vi "x_axisPID_ALB.vi"(6 "First Call?: T/F":bool, 10 "x axis":dbl) -> (2 "x axis out":dbl)   [LabVIEW 2017]
uses:
  <vilib>/addons/control/pid/NI_PID_pid.lvlib
  <vilib>/addons/control/pid/pid.llb/PID (DBL).vi
  <vilib>/addons/control/pid/pid.llb/PID Output Rate Limiter (DBL).vi
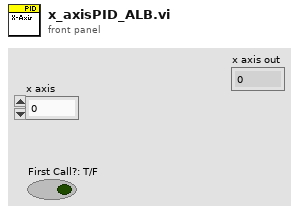
[diagram p1: front panel]
types:
  T1 = cluster{"P":dbl, "I":dbl, "derivative time (Td, min)":dbl}
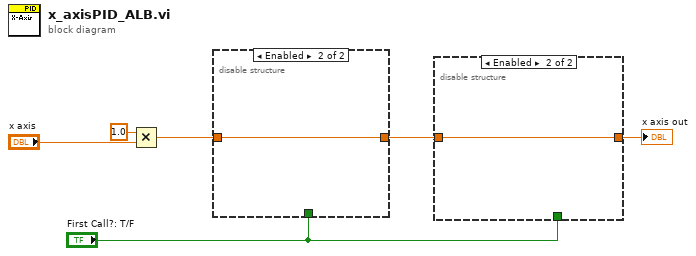
[diagram p0: block diagram]
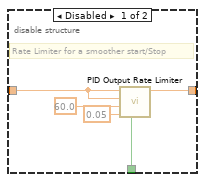
[diagram p2: hidden frame]
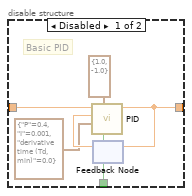
[diagram p3: hidden frame]
diagram:
  n1 = Multiply(x=1.0, y="x axis") -> (x*y=w6:dbl)
  n2 = disable-structure shown="Enabled" {
    disable-tunnel: w6 -> [w12 w13]
    disable-tunnel: [w11 w13] -> w2
    disable-tunnel: "First Call?: T/F" -> [w7 _]
    frame Disabled {
      # "Basic PID"
      n3 = feedback #1() -> (w10:dbl)  [unwired: 1 in]
      n4 = call-poly <vilib>:"PID.vi"("reinitialize? (F)"=w7, "output range"=cluster{"output high":dbl, "output low":dbl} {"output high"=1.0, "output low"=-1.0}, "PID gains"=T1 {"P"=0.4, "I"=0.001, "derivative time (Td, min)"=0.0}, "process variable"=w10, "setpoint"=w12) -> ("output"=w11:dbl)  [unwired: 5 in, 1 out]
      n5 = feedback-in #1(w11) -> ()
    }
    frame Enabled {
    }
  }
  n6 = disable-structure shown="Enabled" {
    disable-tunnel: "First Call?: T/F" -> [w18 _]
    disable-tunnel: w2 -> [w17 w19]
    disable-tunnel: [w15 w19] -> w1
    frame Disabled {
      # "Rate Limiter for a smoother start/Stop"
      n7 = call-poly <vilib>:"PID Output Rate Limiter.vi"("reinitialize? (F)"=w18, "dt (s)"=0.05, "output rate (EGU/min)"=60.0, "initial output"=w17, "input (controller output)"=w17) -> ("output"=w15:dbl)  [unwired: 3 in, 1 out]
    }
    frame Enabled {
    }
  }
  "x axis out" <- w1
